vi "HTTP-Weather.vi"() -> ()   [LabVIEW 2020]
uses:
  <vilib>/httpClient/LabVIEWHTTPClient.lvlib
panel:
  out "see username":string
  in  "password":string
  in  "username":string
  out "Aquired Document":string
  out "URL":string
  in  "longitude":string
  in  "latitude":string
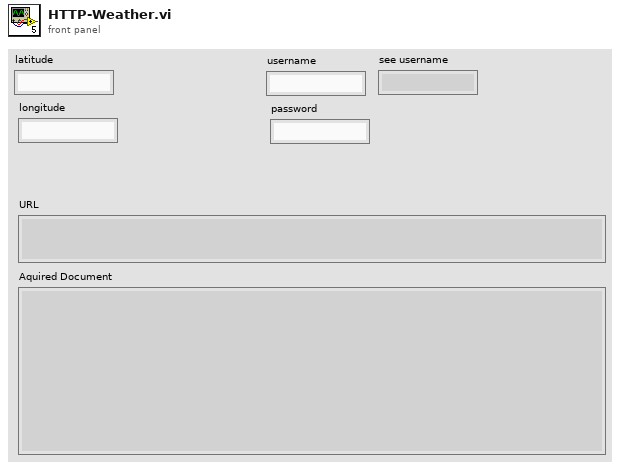
[diagram p1: front panel]
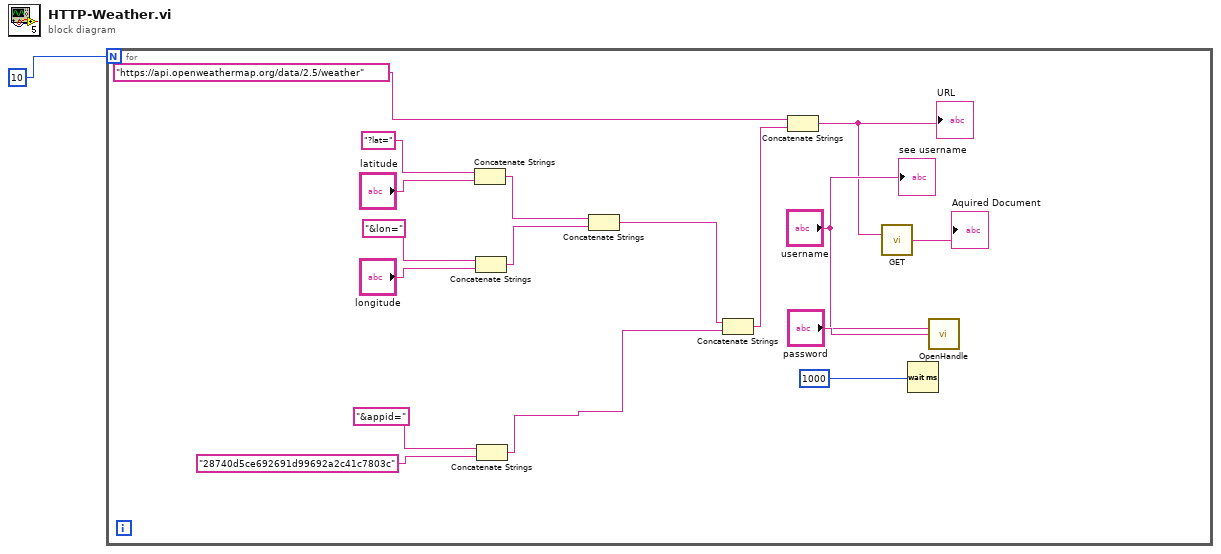
[diagram p0: block diagram]
diagram:
  n1 = for {
    N: 10 -> [_]
    n2 = Concatenate Strings("?lat=", "latitude") -> (w10:string)
    n3 = Concatenate Strings("&lon=", "longitude") -> (w11:string)
    n4 = Concatenate Strings("&appid=", "28740d5ce692691d99692a2c41c7803c") -> (w2:string)
    n5 = Concatenate Strings(w10, w11) -> (w9:string)
    n6 = Concatenate Strings(w9, w2) -> (w8:string)
    n7 = Concatenate Strings("https://api.openweathermap.org/data/2.5/weather", w8) -> (w3:string)
    "URL" <- w3
    n8 = call <vilib>:"GET.vi"("url"=w3) -> ("body"=→"Aquired Document":string)  [unwired: 11 in, 3 out]
    n9 = Wait (ms)(milliseconds to wait=1000) -> ()  [unwired: 1 out]
    n10 = call <vilib>:"OpenHandle.vi"("username"="username", "password"="password") -> ()  [unwired: 12 in, 2 out]
    "see username" <- "username"
  }
